vi "Remove Key.vi"(8 "error in":errorcluster, 10 "Key":string, 11 "E2E configuration in":refnum<class "E2E Tag Exchange configuration.lvclass">) -> (0 "error out":errorcluster, 3 "E2E configuration out":refnum<class "E2E Tag Exchange configuration.lvclass">)   [LabVIEW 2015, in "E2E Tag Exchange configuration.lvclass"]
uses:
  E2E Tag Exchange configuration.lvclass
  E2E Tag Exchange configuration.lvclass/E2E Tag Exchange configuration.ctl
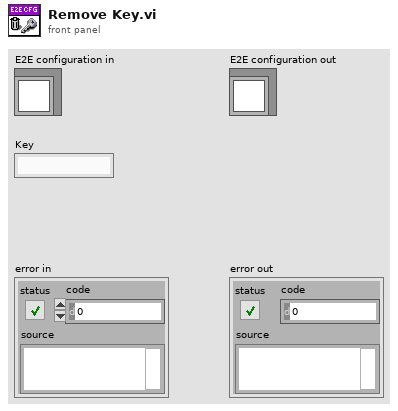
[diagram p1: front panel]
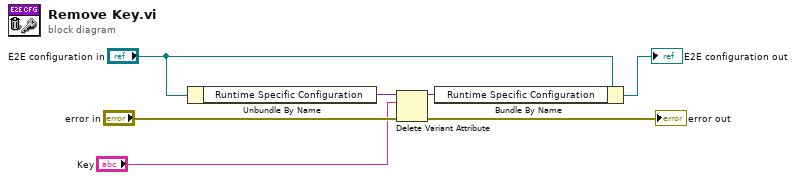
[diagram p0: block diagram]
diagram:
  n1 = Unbundle By Name("E2E configuration in") -> ("Runtime Specific Configuration"=w2:variant)
  n2 = Delete Variant Attribute(4:"error in", 6:"Key", 7:w2) -> (0:→"error out":errorcluster, 3:w6:variant)  [unwired: 1 out]
  n3 = Bundle By Name(cluster="E2E configuration in", "Runtime Specific Configuration"=w6) -> (→"E2E configuration out":refnum<class "E2E Tag Exchange configuration.lvclass">)
